vi "DAQ_LowLevelVI.vi"() -> ()   [LabVIEW 2016]
uses:
  <vilib>/myRIO/Common/Instrument Driver Framework/myRIO v1.0/Encoder/typedefs/Encoder Signal Mode.ctl
  <vilib>/Platform/TimedLoop/XDataNode/timing_clust.ctl
  <vilib>/Platform/TimedLoop/XDataNode/nitl_modes.ctl
  <vilib>/Platform/TimedLoop/XDataNode/wakeup.ctl
  <vilib>/Analysis/3filter.llb/Filter Passband Type.ctl
  <vilib>/myRIO/Common/Instrument Driver Framework/myRIO v1.0/UART/vis/myRIO v1.0 Close UART.vi
  <vilib>/Utility/error.llb/Error Cluster From Error Code.vi
  <vilib>/myRIO/Common/Instrument Driver Framework/myRIO v1.0/Encoder/vis/myRIO v1.0 Read Encoder.vi
  <vilib>/myRIO/Common/Instrument Driver Framework/myRIO v1.0/AI/vis/myRIO v1.0 Read AI.vi
  <vilib>/Analysis/3filter.llb/Butterworth Filter (DBL).vi
  <vilib>/myRIO/Common/Instrument Driver Framework/Utilities/vis/FPGA Ref Manager.vi
  <vilib>/myRIO/Common/Instrument Driver Framework/myRIO v1.0/myRIO v1.0 Reset FPGA.vi
  <vilib>/myRIO/Common/Instrument Driver Framework/myRIO v1.0/IRQ/vis/myRIO v1.0 IRQ Info FGV.vi
  <vilib>/myRIO/Common/Instrument Driver Framework/myRIO v1.0/IRQ/vis/myRIO v1.0 Timer IRQ Info FGV.vi
  <vilib>/myRIO/Common/Instrument Driver Framework/myRIO v1.0/IRQ/vis/myRIO v1.0 ISR Agent.vi
  <vilib>/Platform/TimedLoop/XDataNode/XDataNode.xnode
  <vilib>/myRIO/Instrument Drivers/Onboard IO/Encoder/Encoder.lvlib
  <vilib>/myRIO/Instrument Drivers/Onboard IO/AI/AI.lvlib
  <vilib>/myRIO/Instrument Drivers/Utilities/Utilities.lvlib
  <vilib>/Platform/TimedLoop/XDataNode/XDNodeRunTimeDep.lvlib
  <vilib>/Analysis/NI_AALBase.lvlib
panel:
  out "L Heel (V)":dbl(slide) scale=0.0..2.0
  out "L 1st Meta (V)":dbl(slide) scale=0.0..2.0
  out "L Toe (V) 2":dbl(slide) scale=0.0..2.0
  out "Joint_Enc_L":i32
  out "Toe (V)":dbl(slide) scale=0.0..2.0
  out "1st Meta (V)":dbl(slide) scale=0.0..2.0
  out "Heel (V)":dbl(slide) scale=0.0..2.0
  out "Spring (V)":dbl
  out "Mtr_2 (rpm)":i32
  out "Mtr_1 (rpm)":i32
  out "Spring (N)":dbl
  out "Fd (N)":dbl(knob) scale=-100.0..100.0
  out "Fp (N)":dbl(knob) scale=-100.0..100.0
  out "Joint_Enc_R":i32
  out "Late?":bool
  in  "stop 3":bool
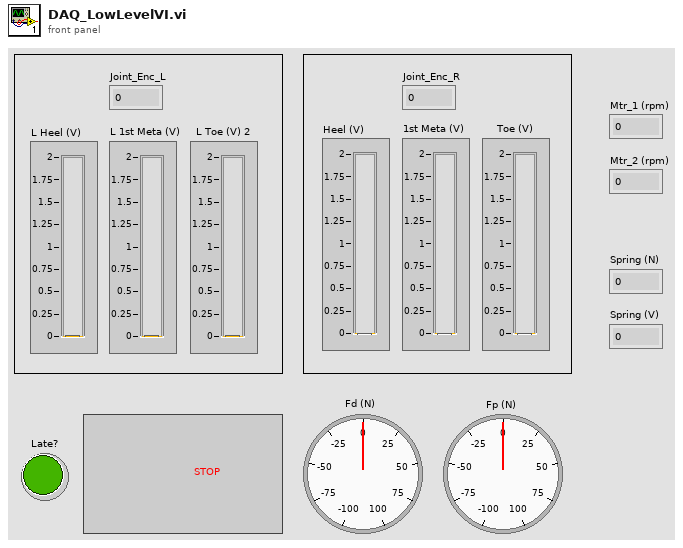
[diagram p1: front panel]
types:
  T1 = typedef "Encoder Signal Mode.ctl" = enum16{"Quadrature phase signal", "Step and direction signal"}
  T2 = typedef "Encoder.lvlib/Encoder Reference.ctl" = cluster{"myRIO Reference":T3, "Encoder Channels Enum":T7}
  T3 = typedef "myRIO Generic Hardware Reference.ctl" = cluster{"myRIO Model":T4, "myRIO Hardware Reference":T5}
  T4 = typedef "Hardware Version Enum.ctl" = enum16{"Unknown", "myRIO-1900", "myRIO-1950", "roboRIO", "NI ELVIS RIO CM"}
  T5 = typedef "myRIO v1.0 Reference.ctl" = cluster{"Generic FPGA Reference":T6, "Allow multiple opens":bool}
  T6 = typedef "Generic FPGA Reference.ctl" = refnum<k20>
  T7 = typedef "Encoder Channels Enum.ctl" = enum16{"Not Connected", "C/ENC0", "C/ENC1", "A/ENC", "B/ENC", "DIO/ENC0", "DIO/ENC1", "DIO/ENC2", "DIO/ENC3", "DIO/ENC4"}
  T8 = typedef "AI.lvlib/AI Reference.ctl" = cluster{"myRIO Reference":T3, "AI Channels List":T9, "AI Scaling Constants List":T11}
  T9 = typedef "AI Channels List.ctl" = T10[]
  T10 = typedef "AI Channels Enum.ctl" = enum16{"Not Connected", "AudioIn/Left", "AudioIn/Right", "C/AI0", "C/AI1", "A/AI0", "A/AI1", "A/AI2", "A/AI3", "B/AI0", "B/AI1", "B/AI2", "B/AI3", "AI/AI0", "AI/AI1", "AI/AI2", "AI/AI3"}
  T11 = typedef "Analog Scaling Constants List.ctl" = T12[]
  T12 = typedef "Analog Scaling Constants.ctl" = cluster{"LSB Weight (Volts)":dbl, "Offset (Volts)":dbl, "Signed?":bool}
  T13 = typedef "XDNodeRunTimeDep.lvlib/timing_clust.ctl" = cluster{"Expected End [f-1]":u64, "Actual End [f-1]":u64, "Finished Late? [f-1]":bool, "Expected End [i-1]":u64, "Actual End [i-1]":u64, "Finished Late? [i-1]":bool, "Expected Start [i]":u64, "Actual Start [i]":u64, "Expected Start [f]":u64, "Actual Start [f]":u64, "Source Name":string, "Structure Name":string, "Period":i64, "Deadline":i64, "Offset":i64, "Start":i64, "Priority":i32, "Timeout":i32, "Mode":T14, "Wakeup Reason":T15, "Error":errorcluster, "Source Type":string, "Secondary Source Type":string, "Global End Time":u64, "Global Start Time":u64, "Frame Duration":u64, "Iteration Duration":u64, "Assigned CPU":i32, "I/O Scan Engine Mode":u32}
  T14 = typedef "XDNodeRunTimeDep.lvlib/nitl_modes.ctl" = enum32{"No Change", "Process missed periods, maintain original phase", "Discard missed periods, maintain original phase", "Process missed periods, ignore original phase", "Discard missed periods, ignore original phase"}
  T15 = typedef "XDNodeRunTimeDep.lvlib/wakeup.ctl" = enum32{"Normal", "Aborted", "Asynchronous wakeup", "Timing source error", "Timed loop error", "Timeout"}
  T16 = typedef "NI_AALBase.lvlib/Filter Passband Type.ctl" = enum32{"Lowpass", "Highpass", "Bandpass", "Bandstop"}
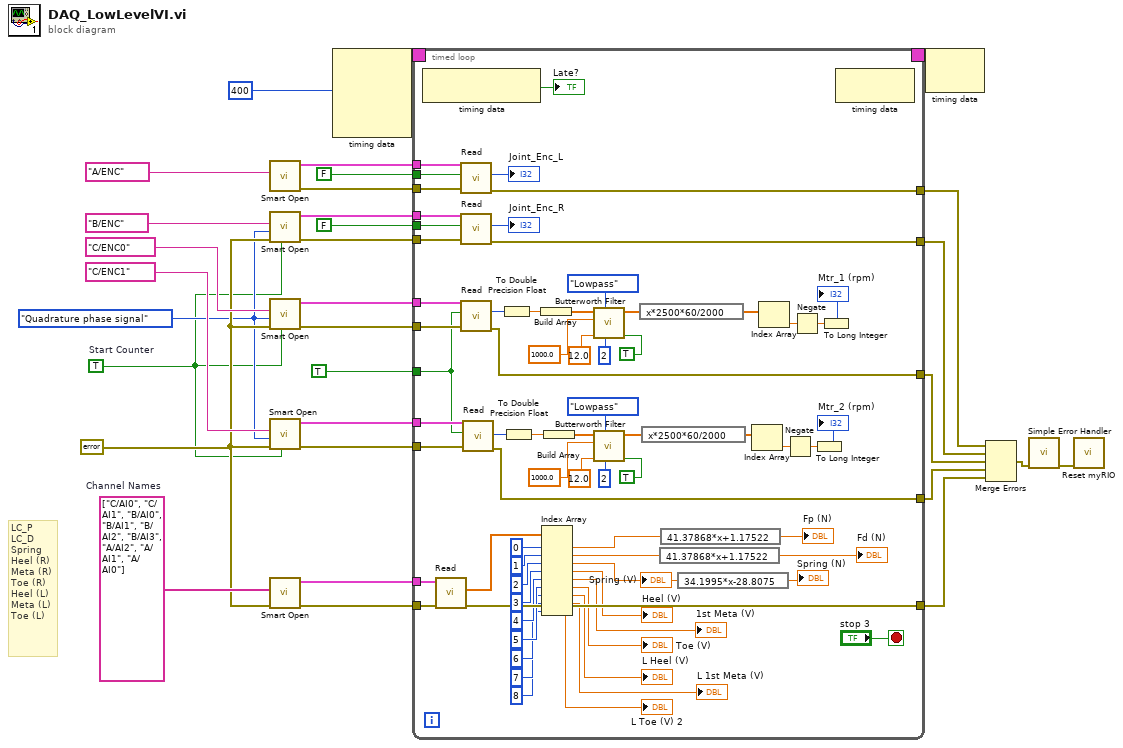
[diagram p0: block diagram]
diagram:
  w19 = errorcluster {"status"=FALSE, "code"=0, "source"=""} ("error in (no error)")
  w20 = tag[] ["C/AI0", "C/AI1", "B/AI0", "B/AI1", "B/AI2", "B/AI3", "A/AI2", "A/AI1", "A/AI0"]  # Channel Names
  w10 = TRUE  # Start Counter
  w11 = Encoder_Signal_Mode."Quadrature phase signal" ("Encoder Signal Mode")
  # "LC_P\nLC_D\nSpring\nHeel (R)\nMeta (R)\nToe (R)\nHeel (L)\nMeta (L)\nToe (L)"
  n1 = call <vilib>:"Smart Open.vi"("Channel Name"=tag "A/ENC") -> ("error out"=w2:errorcluster, "Encoder Ref Out"=w3:T2)  [unwired: 9 in]
  n2 = call <vilib>:"Smart Open.vi"("Start Counter"=w10, "error in (no error)"=w19, "Encoder Signal Mode"=w11, "Channel Name"=tag "B/ENC") -> ("error out"=w27:errorcluster, "Encoder Ref Out"=w28:T2)  [unwired: 6 in]
  n3 = call <vilib>:"Smart Open.vi"("Start Counter"=w10, "error in (no error)"=w19, "Encoder Signal Mode"=w11, "Channel Name"=tag "C/ENC0") -> ("error out"=w26:errorcluster, "Encoder Ref Out"=w25:T2)  [unwired: 6 in]
  n4 = call <vilib>:"Smart Open.vi"("Start Counter"=w10, "error in (no error)"=w19, "Encoder Signal Mode"=w11, "Channel Name"=tag "C/ENC1") -> ("error out"=w21:errorcluster, "Encoder Ref Out"=w22:T2)  [unwired: 6 in]
  n5 = call <vilib>:"Smart Open.vi"("error in (no error)"=w19, "Channel Names"=w20) -> ("error out"=w17:errorcluster, "AI Ref Out"=w18:T8)  [unwired: 8 in]
  n6 = node-c288(i64 400 ("Period")) -> (w31:T13)  [unwired: 3 in]
  n7 = timed-loop {
    tunnel: w28 -> [w100]
    tunnel: w27 -> [w99]
    tunnel: w25 -> [w97]
    tunnel: w26 -> [w98]
    tunnel: w22 -> [w96]
    tunnel: w21 -> [w95]
    tunnel: w18 -> [w93]
    tunnel: w17 -> [w92]
    tunnel: [w91] -> w14
    tunnel: [w84] -> w13
    tunnel: [w90] -> w12
    timing: w31 -> [_]
    timing-out: [_] -> w30
    tunnel: [w85] -> w8
    tunnel: TRUE ("Reset Counter") -> [w52]
    tunnel: FALSE ("Reset Counter") -> [w51]
    tunnel: FALSE ("Reset Counter") -> [w42]
    tunnel: w3 -> [w41]
    tunnel: w2 -> [w40]
    tunnel: [w38] -> w1
    stop <- "stop 3" stop-if-true
    n8 = node-c288() -> (→"Late?":bool)  [unwired: 1 in]
    n9 = call <vilib>:"Read.vi"("error in (no error)"=w92, "AI Ref In"=w93) -> ("error out"=w90:errorcluster, "Values"=w94:dbl[])  [unwired: 7 in, 1 out]
    n10 = call <vilib>:"Read.vi"("error in (no error)"=w40, "Reset Counter"=w42, "Encoder Ref In"=w41) -> ("error out"=w38:errorcluster, "Counter Value"=→"Joint_Enc_L":i32)  [unwired: 4 in, 3 out]
    n11 = call <vilib>:"Read.vi"("error in (no error)"=w99, "Reset Counter"=w51, "Encoder Ref In"=w100) -> ("error out"=w91:errorcluster, "Counter Value"=→"Joint_Enc_R":i32)  [unwired: 4 in, 3 out]
    n12 = call <vilib>:"Read.vi"("error in (no error)"=w98, "Reset Counter"=w52, "Encoder Ref In"=w97) -> ("error out"=w85:errorcluster, "Counter Value"=w70:i32)  [unwired: 4 in, 3 out]
    n13 = call <vilib>:"Read.vi"("error in (no error)"=w95, "Reset Counter"=w52, "Encoder Ref In"=w96) -> ("error out"=w84:errorcluster, "Counter Value"=w57:i32)  [unwired: 4 in, 3 out]
    n14 = To Double Precision Float(number=w70) -> (double precision float=w69:dbl)
    n15 = To Double Precision Float(number=w57) -> (double precision float=w66:dbl)
    n16 = Build Array(w69) -> (w68:dbl[])
    n17 = Index Array(array=w94, index #1=0 ("index"), index #2=1 ("index"), index #3=2 ("index"), index #4=3 ("index"), index #5=4 ("index"), index #6=5 ("index"), index #7=6 ("index"), index #8=7 ("index"), index #9=8 ("index")) -> (element #1=w81:dbl, element #2=w82:dbl, element #3=w49:dbl, element #4=→"Heel (V)":dbl, element #5=→"1st Meta (V)":dbl, element #6=→"Toe (V)":dbl, element #7=→"L Heel (V)":dbl, element #8=→"L 1st Meta (V)":dbl, element #9=→"L Toe (V) 2":dbl)
    "Spring (V)" <- w49
    n18 = Build Array(w66) -> (w67:dbl[])
    n19 = call-poly <vilib>:"Butterworth Filter.vi"("init/cont (init:F)"=TRUE, "order"=2, "filter type"=Filter_Passband_Type."Lowpass", "low cutoff freq: fl"=12.0, "sampling freq: fs"=1000.0, "X"=w68) -> ("Filtered X"=w73:dbl[])  [unwired: 2 in, 1 out]
    n20 = call-poly <vilib>:"Butterworth Filter.vi"("init/cont (init:F)"=TRUE, "order"=2, "filter type"=Filter_Passband_Type."Lowpass", "low cutoff freq: fl"=12.0, "sampling freq: fs"=1000.0, "X"=w67) -> ("Filtered X"=w63:dbl[])  [unwired: 2 in, 1 out]
    n21 = expression code="x*2500*60/2000"(w73) -> (w72:dbl[])
    n22 = expression code="x*2500*60/2000"(w63) -> (w64:dbl[])
    n23 = expression code="41.37868*x+1.17522"(w82) -> (→"Fd (N)":dbl)
    n24 = expression code="41.37868*x+1.17522"(w81) -> (→"Fp (N)":dbl)
    n25 = expression code="34.1995*x-28.8075"(w49) -> (→"Spring (N)":dbl)
    n26 = Index Array(array=w64) -> (element=w65:dbl)  [unwired: 1 in]
    n27 = Index Array(array=w72) -> (element=w71:dbl)  [unwired: 1 in]
    n28 = Negate(x=w65) -> (-x=w54:dbl)
    n29 = Negate(x=w71) -> (-x=w56:dbl)
    n30 = To Long Integer(number=w54) -> (32bit integer=→"Mtr_2 (rpm)":i32)
    n31 = To Long Integer(number=w56) -> (32bit integer=→"Mtr_1 (rpm)":i32)
    n32 = node-c288() -> ()  [unwired: 1 in, 1 out]
  }
  n33 = node-c288(w30) -> ()  [unwired: 1 out]
  n34 = Merge Errors(w1, w14, w8, w13, w12) -> (w16:errorcluster)
  n35 = call <vilib>:"Simple Error Handler.vi"("error in (no error)"=w16) -> ("error out"=w15:errorcluster)  [unwired: 4 in, 4 out]
  n36 = call <vilib>:"Reset myRIO.vi"("error in (no error)"=w15) -> ()  [unwired: 10 in, 1 out]
